vi "dlugosc_odczytanego_slowa.vi"() -> ()   [LabVIEW 2018]
panel:
  in  "Ile czytac":i32
  out "Status":bool
  in  "ile szukasz":i32
  out "error out":errorcluster
  in  "file path (use dialog)":path
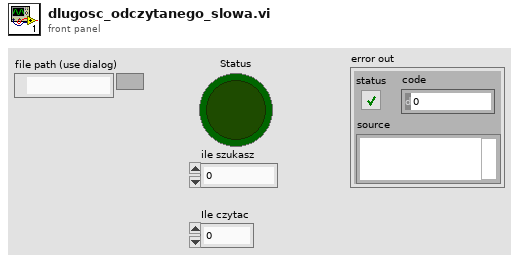
[diagram p1: front panel]
types:
  T1 = enum16{"open", "replace", "create", "open or create", "replace or create", "replace or create with confirmation"}
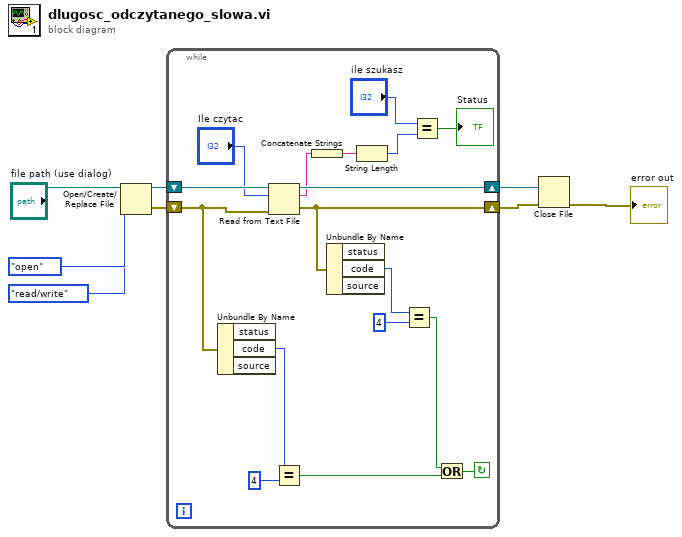
[diagram p0: block diagram]
diagram:
  n1 = Open/Create/Replace File(file path (use dialog)="file path (use dialog)", operation (0:open)=T1."open", access (0:read/write)=enum16{"read/write", "read-only", "write-only"}."read/write") -> (refnum out=w5:refnum<file>, error out=w2:errorcluster)  [unwired: 3 in, 1 out]
  n2 = while {
    shift-right: [w24] -> w4
    shift-left: w5 -> [w25]
    shift-right: [w14] -> w3
    shift-left: w2 -> [w19]
    stop <- w9 continue-if-true
    n3 = Unbundle By Name(w19) -> ("code"=w18:i32)  [unwired: 2 out]
    n4 = Read from Text File(file (use dialog)=w25, count="Ile czytac", error in=w19) -> (refnum out=w24:refnum<file>, text=w20:string, error out=w14:errorcluster)  [unwired: 1 in, 1 out]
    n5 = Equal?(x=w18, y=4) -> (x = y?=w10:bool)
    n6 = Concatenate Strings(w20) -> (w15:string)
    n7 = Unbundle By Name(w14) -> ("code"=w13:i32)  [unwired: 2 out]
    n8 = String Length(string=w15) -> (length=w16:i32)
    n9 = Equal?(x=w13, y=4) -> (x = y?=w11:bool)
    n10 = Equal?(x="ile szukasz", y=w16) -> (x = y?=→"Status":bool)
    n11 = Or(x=w11, y=w10) -> (x .or. y?=w9:bool)
  }
  n12 = Close File(refnum=w4, error in=w3) -> (error out=→"error out":errorcluster)  [unwired: 1 out]
